vi "FFController_GetForce.vi"(8 "error in (no error)":errorcluster, 11 "Force Field Controller in":refnum<class "Force Field Controller.lvclass">) -> (0 "error out":errorcluster, 2 "Force":dbl[](array[numeric]), 3 "Force Field Controller out":refnum<class "Force Field Controller.lvclass">)   [LabVIEW 2012, in "Force Field Controller.lvclass"]
uses:
  Force Field Controller.lvclass
  Force Field Controller.lvclass/Force Field Controller.ctl
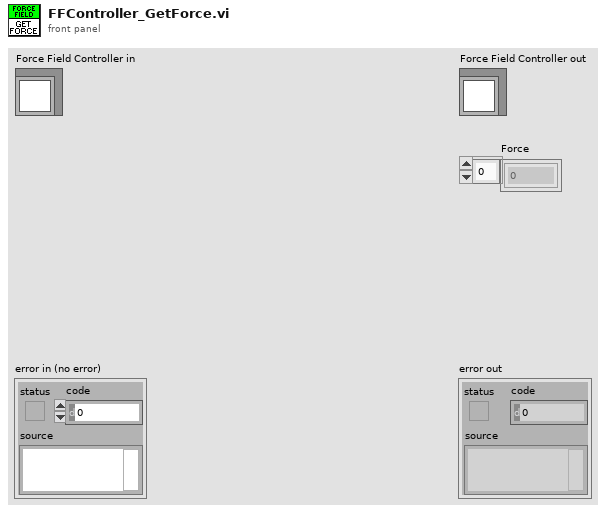
[diagram p1: front panel]
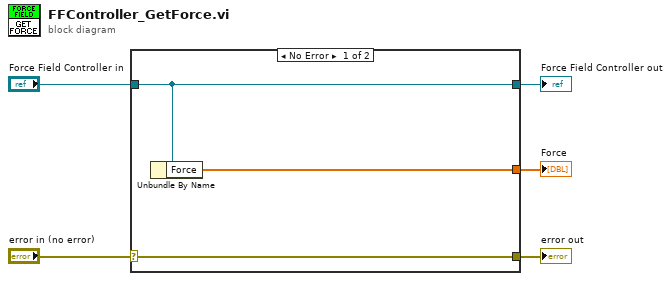
[diagram p0: block diagram]
diagram:
  n1 = case shown="No Error" "error in (no error)" {
    selector: "error in (no error)" -> [w8 w9]
    tunnel: [w8 w9] -> w4
    tunnel: [w7 w10] -> w2
    tunnel: "Force Field Controller in" -> [w7 w10]
    tunnel: [w6 _] -> w1
    frame No Error {
      n2 = Unbundle By Name(w7) -> ("Force"=w6:dbl[])
    }
    frame Error {
    }
  }
  "error out" <- w4
  "Force Field Controller out" <- w2
  "Force" <- w1
